vi "Set_Json_Parameter.vi"(8 "error in (no error)":errorcluster caption="entrée d'erreur (pas d'erreur)", 10 "Json_Parameter":string, 11 "Popup Autotest (Default) en entrée":refnum<class "Popup Autotest (Default).lvclass">) -> (0 "error out":errorcluster caption="sortie d'erreur", 3 "Popup Autotest (Default) en sortie":refnum<class "Popup Autotest (Default).lvclass">)   [LabVIEW 2020, in "Library Instrument & Equipement.lvlib" / "Library Popup.lvlib" / "Popup Autotest (Default).lvclass"]
uses:
  Popup Autotest (Default).lvclass
  Class Popup (Main)/Class Popup (Main).lvclass
  Popup Autotest (Default).lvclass/Popup Autotest (Default).ctl
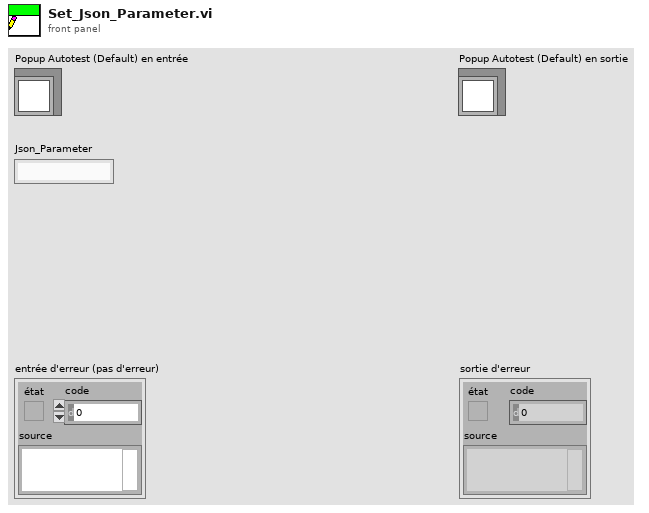
[diagram p1: front panel]
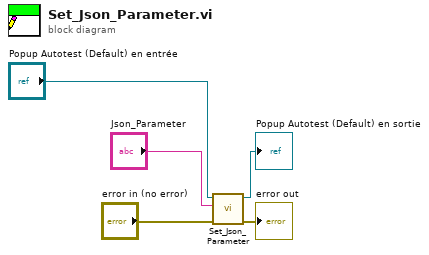
[diagram p0: block diagram]
diagram:
  n1 = call-parent "Set_Json_Parameter.vi"("error in (no error)"="error in (no error)", "Json_Parameter"="Json_Parameter", "Class Popup (Main) en entrée"="Popup Autotest (Default) en entrée") -> ("error out"=→"error out":errorcluster, "Class Popup (Main) en sortie"=→"Popup Autotest (Default) en sortie":refnum<class "Popup Autotest (Default).lvclass">)  [unwired: 7 in]
